vi "GetContextHelpInfo.vi"(0 "reference":refnum<class "ClassRelationshipEdge.lvclass">, 1 "MousePos":T1 {"y" format="%.2f"; "x" format="%.2f"}, 5 "error in (no error)":errorcluster) -> (14 "reference out":refnum<class "ClassRelationshipEdge.lvclass">, 15 "ContextHelpInfoExist":bool, 16 "ContextHelpInfo":variant, 17 "Rows":string[](array[string]), 19 "error out":errorcluster)   [LabVIEW 2014, in "ClassRelationshipEdge.lvclass"]
doc: "GetContextHelpInfo"
uses:
  <resource>/Framework/Providers/Open_GDS/UML/ClassRelationshipEdge_class/ClassRelationshipEdge.lvclass
  <resource>/Framework/Providers/Open_GDS/UML/General/Point/Point Point2D.ctl
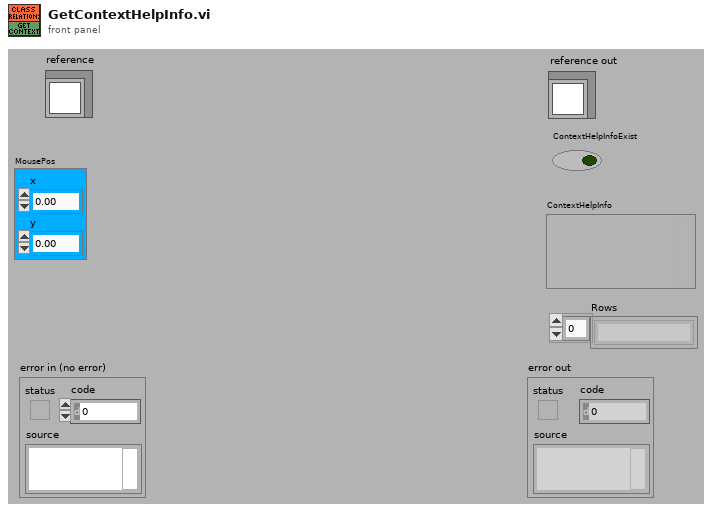
[diagram p1: front panel]
types:
  T1 = typedef "Point Point2D.ctl" = cluster{"x":dbl, "y":dbl}
  T2 = typedef "ClassRelationshipEdge.lvclass/ObjectAttributes.ctl" = cluster{"bentStyleRef":refnum<class "BentStyle.lvclass">, "startConnectionOffset":cluster{"x":i32, "y":i32}, "endConnectionOffset":cluster{"x":i32, "y":i32}, "MidLineOffset":cluster{"x":i32, "y":i32}, "DepClass":T3}
  T3 = typedef "ReversedEngineering_ViDependencyDetailsType.ctl" = cluster{"ThisVIs/Ctls":path[], "Dependent_VIs/Ctls":path[]}
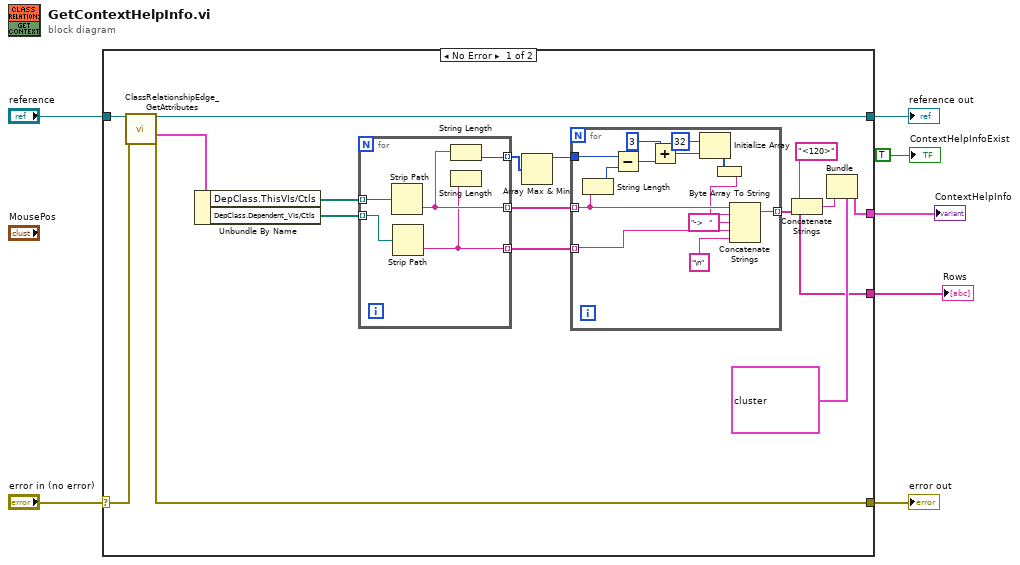
[diagram p0: block diagram]
diagram:
  n1 = case shown="No Error" "error in (no error)" {
    selector: "error in (no error)" -> [w23 w42]
    tunnel: "reference" -> [w22 w43]
    tunnel: [w20 w42] -> w5
    tunnel: [w21 w43] -> w4
    tunnel: [w11 _] -> w3
    tunnel: [w10 _] -> w1
    frame No Error {
      n2 = call <resource>:"ClassRelationshipEdge_GetAttributes.vi"("reference in"=w22, "error in (no error)"=w23) -> ("reference out"=w21:refnum<class "ClassRelationshipEdge.lvclass">, "Data"=w8:T2, "error out"=w20:errorcluster)  [unwired: 1 in, 14 out]
      n3 = Unbundle By Name(w8) -> ("DepClass.ThisVIs/Ctls"=w19:path[], "DepClass.Dependent_VIs/Ctls"=w18:path[])
      n4 = for {
        tunnel: w19 -> [w41] mode=indexing
        tunnel: w18 -> [w40] mode=indexing
        tunnel: [w37] -> w15 mode=indexing
        tunnel: [w39] -> w17 mode=indexing
        tunnel: [w38] -> w16 mode=indexing
        n5 = Strip Path(path=w41) -> (name=w39:string)  [unwired: 1 out]
        n6 = Strip Path(path=w40) -> (name=w38:string)  [unwired: 1 out]
        n7 = String Length(string=w39) -> (length=w37:i32)
        n8 = String Length(string=w38) -> ()  [unwired: 1 out]
      }
      n9 = Array Max & Min(array=w15) -> (max value=w14:i32)  [unwired: 3 out]
      n10 = for {
        tunnel: w17 -> [w29] mode=indexing
        tunnel: w16 -> [w26] mode=indexing
        tunnel: w14 -> [w35]
        tunnel: [w27] -> w10 mode=indexing
        n11 = String Length(string=w29) -> (length=w36:i32)
        n12 = Subtract(x=w35, y=w36) -> (x-y=w34:i32)
        n13 = Add(x=3, y=w34) -> (x+y=w32:i32)
        n14 = Initialize Array(u8 32 ("element"), w32) -> (w30:u8[])
        n15 = Byte Array To String(unsigned byte array=w30) -> (string=w28:string)
        n16 = Concatenate Strings(w29, w28, "->   " ("string"), w26, "\n") -> (w27:string)
      }
      n17 = Concatenate Strings("<120>", w10) -> (w13:string)
      n18 = Bundle(cluster=cluster{string, "empty picture":picture, string} {"Dependencies", "empty picture"=bytes[0], ""}, w13) -> (w11:cluster{string, "empty picture":picture, string})  [unwired: 2 out]
    }
    frame Error {
    }
  }
  "reference out" <- w4
  "error out" <- w5
  "ContextHelpInfo" <- w3
  "Rows" <- w1
  "ContextHelpInfoExist" <- TRUE ("ContextHelpInfoExist")
